vi "Set Name.vi"(7 "Tree ID":string, 8 "Error In":errorcluster, 10 "Name":string, 11 "Tree Manager":T1) -> (0 "Error Out":errorcluster, 3 "Tree Manager":T1)   [LabVIEW 2016, in "Tree Manager.lvclass"]
doc: "Set the Name of the Tree."
uses:
  Tree Manager.lvclass
  Typedefs/Session Handle.ctl
  Tree Manager.lvclass/Tree Manager.ctl
  Typedefs/Tree.ctl
  <vilib>/Utility/error.llb/Error Cluster From Error Code.vi
  <vilib>/ErrorRing/Error Ring.xnode
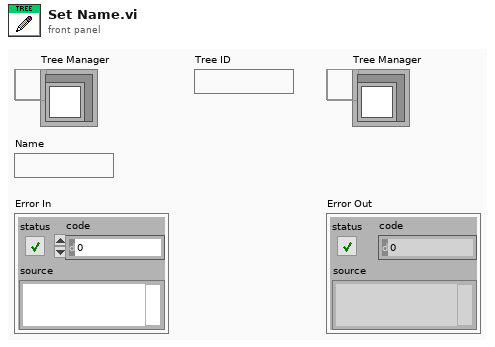
[diagram p1: front panel]
types:
  T1 = typedef "Tree Manager.lvclass/Session Handle.ctl" = refnum<data-value>
  T2 = typedef "Tree Manager.lvclass/Tree.ctl" = cluster{"Unique ID":string, "Parent ID":string, "Child IDs":string[], "Data":variant, "Name":string}
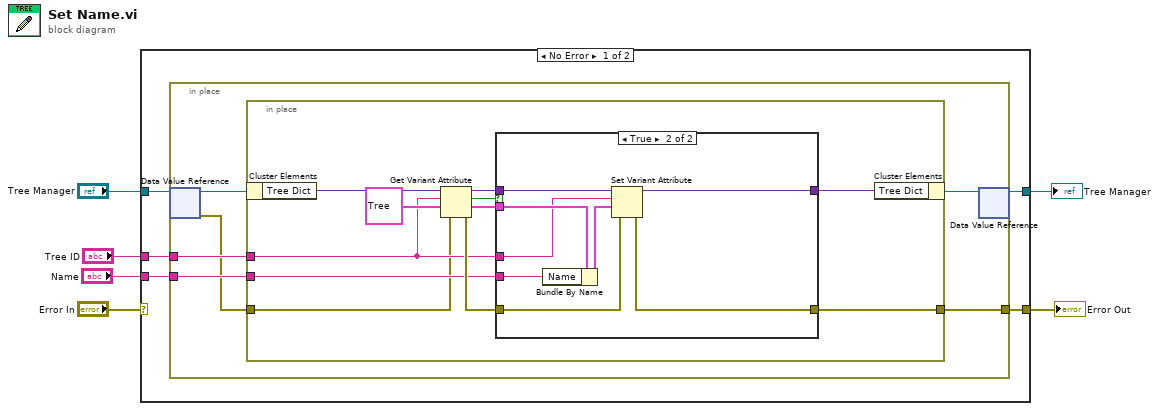
[diagram p0: block diagram]
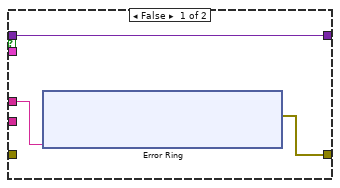
[diagram p2: hidden frame]
diagram:
  n1 = case shown="No Error" "Error In" {
    selector: "Error In" -> [_ w47]
    tunnel: "Tree Manager" -> [w11 w48]
    tunnel: [w10 w48] -> w5
    tunnel: [w9 w47] -> w3
    tunnel: "Tree ID" -> [w8 _]
    tunnel: "Name" -> [w7 _]
    frame No Error {
      n2 = in-place {
        in-place-border: [w16] -> w9
        in-place-border: w8 -> [w14]
        in-place-border: w7 -> [w13]
        n3 = in-place-dvr #1(w11) -> (w17:refnum<class "Tree Manager.lvclass">, w12:errorcluster)
        n4 = in-place {
          in-place-border: [w18] -> w16
          in-place-border: w12 -> [w19]
          in-place-border: w14 -> [w21]
          in-place-border: w13 -> [w20]
          n5 = in-place-cluster #2(w17) -> ("Tree Dict"=w24:variant)
          n6 = Get Variant Attribute(Variant=w24, name=w21, default value (empty Variant)=T2 {"Unique ID"="", "Parent ID"="", "Child IDs"=[], "Data"=variant, "Name"=""} ("Cluster of class private data"), error in=w19) -> (duplicate Variant=w27:variant, found=w25:bool, value=w26:T2, error out=w28:errorcluster)
          n7 = case shown="True" w25 {
            tunnel: w26 -> [_ w42]
            tunnel: w27 -> [w31 w46]
            tunnel: w28 -> [_ w43]
            tunnel: [w30 w44] -> w18
            tunnel: [w31 w45] -> w23
            tunnel: w21 -> [w29 w40]
            tunnel: w20 -> [_ w39]
            frame False {
              n8 = xnode "Error Ring"("parameter 0"=w29) -> ("error out"=w30:errorcluster)
            }
            frame True {
              n9 = Bundle By Name(cluster=w42, "Name"=w39) -> (w41:T2)
              n10 = Set Variant Attribute(Variant=w46, name=w40, value=w41, error in=w43) -> (Variant out=w45:variant, error out=w44:errorcluster)  [unwired: 1 out]
            }
          }
          n11 = in-place-cluster #2("Tree Dict"=w23) -> (w15:refnum<class "Tree Manager.lvclass">)
        }
        n12 = in-place-dvr #1(w15) -> (w10:T1)  [unwired: 1 out]
      }
    }
    frame Error {
    }
  }
  "Tree Manager" <- w5
  "Error Out" <- w3
